vi "Y_profile_triangle_adjustable.vi"(2 "FF frame in?":bool, 3 "y resolution":u16, 4 "Vy min(bits)":i16, 5 "y step size":u16, 6 "line counter":u16) -> (0 "FF frame out?":bool, 1 "y signal":i16)   [LabVIEW 2010]
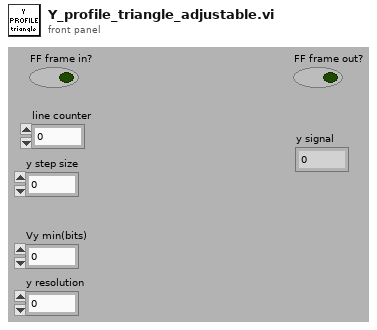
[diagram p1: front panel]
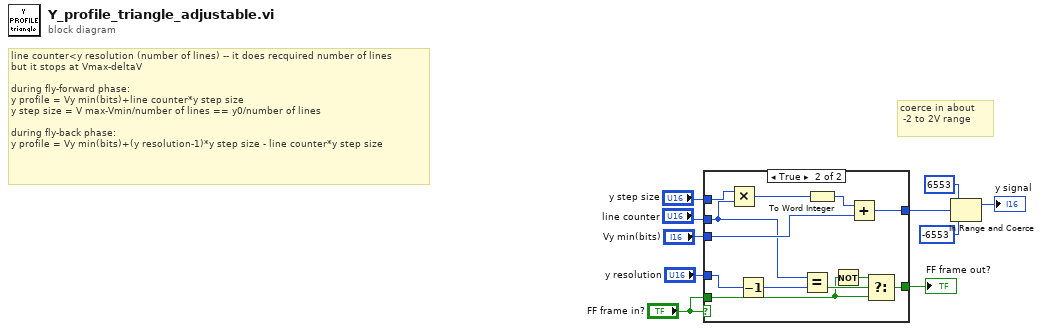
[diagram p0: block diagram]
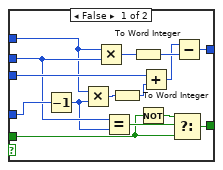
[diagram p2: hidden frame]
diagram:
  # "coerce in about\n -2 to 2V range"
  # "line counter<y resolution (number of lines) -- it does recquired number of lines\nbut it stops at Vmax-deltaV\n\nduring fly-forward phase:\ny profile = Vy min(bits)+line counter*y step size\ny step size = V max-Vmin/number of lines == y0/number of lines\n\nduring fly-back phase:\ny profile = Vy min(bits)+(y resolution-1)*y step size - line counter*y step size"
  n1 = case shown="True" "FF frame in?" {
    tunnel: "y step size" -> [w12 w37]
    tunnel: "line counter" -> [w15 w32]
    tunnel: "Vy min(bits)" -> [w23 w35]
    tunnel: [w16 w29] -> w5
    tunnel: "FF frame in?" -> [w14 w28]
    tunnel: "y resolution" -> [w22 w31]
    tunnel: [w13 w26] -> w1
    frame False {
      n2 = Decrement(x=w22) -> (x-1=w11:u16)
      n3 = Multiply(x=w12, y=w11) -> (x*y=w24:u16)
      n4 = Multiply(x=w12, y=w15) -> (x*y=w25:u16)
      n5 = Equal?(x=w15, y=w11) -> (x = y?=w18:bool)
      n6 = To Word Integer(number=w24) -> (16bit integer=w21:i16)
      n7 = To Word Integer(number=w25) -> (16bit integer=w20:i16)
      n8 = Not(x=w14) -> (.not. x?=w17:bool)
      n9 = Add(x=w23, y=w21) -> (x+y=w19:i16)
      n10 = Select(t=w17, s=w18, f=w14) -> (s? t:f=w16:bool)
      n11 = Subtract(x=w19, y=w20) -> (x-y=w13:i16)
    }
    frame True {
      n12 = Multiply(x=w37, y=w32) -> (x*y=w34:u16)
      n13 = Decrement(x=w31) -> (x-1=w30:u16)
      n14 = Equal?(x=w32, y=w30) -> (x = y?=w33:bool)
      n15 = To Word Integer(number=w34) -> (16bit integer=w36:i16)
      n16 = Not(x=w28) -> (.not. x?=w27:bool)
      n17 = Add(x=w36, y=w35) -> (x+y=w26:i16)
      n18 = Select(t=w27, s=w33, f=w28) -> (s? t:f=w29:bool)
    }
  }
  "FF frame out?" <- w5
  n19 = In Range and Coerce(upper limit=i16 6553, x=w1, lower limit=i16 -6553) -> (coerced(x)=→"y signal":i16)  [unwired: 1 out]
